vi "Output Current(SubVI).vi"(4 "I_sh":dbl, 5 "V":dbl, 6 "I_0":dbl, 7 "R_s":dbl, 8 "n":dbl, 9 "T":dbl, 10 "I_ph":dbl, 11 "N_s":dbl) -> (3 "I":dbl)   [LabVIEW 2024]
panel:
  in  "I_1":dbl
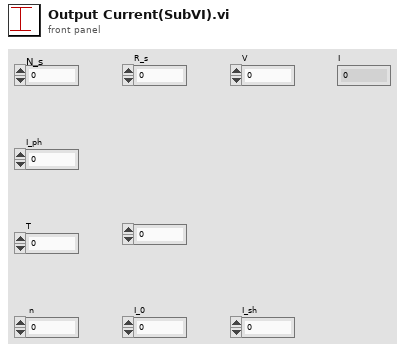
[diagram p1: front panel]
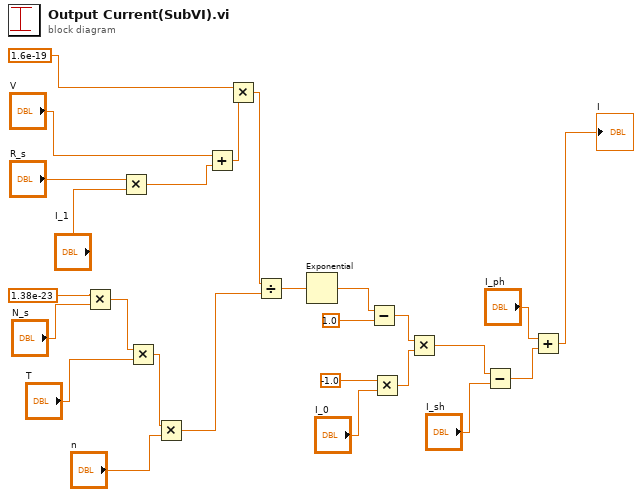
[diagram p0: block diagram]
diagram:
  n1 = Multiply(x=1.38e-23, y="N_s") -> (x*y=w5:dbl)
  n2 = Multiply(x="R_s", y="I_1") -> (x*y=w12:dbl)
  n3 = Multiply(x=w5, y="T") -> (x*y=w8:dbl)
  n4 = Multiply(x=w8, y="n") -> (x*y=w9:dbl)
  n5 = Add(x="V", y=w12) -> (x+y=w13:dbl)
  n6 = Multiply(x=1.6e-19, y=w13) -> (x*y=w15:dbl)
  n7 = Divide(x=w15, y=w9) -> (x/y=w23:dbl)
  n8 = Exponential(1:w23) -> (0:w25:dbl)
  n9 = Subtract(x=w25, y=1.0) -> (x-y=w26:dbl)
  n10 = Multiply(x=-1.0, y="I_0") -> (x*y=w18:dbl)
  n11 = Multiply(x=w26, y=w18) -> (x*y=w19:dbl)
  n12 = Subtract(x=w19, y="I_sh") -> (x-y=w21:dbl)
  n13 = Add(x="I_ph", y=w21) -> (x+y=→"I":dbl)
